vi "basic read field.vi"() -> (2 "Field":dbl[unit])   [LabVIEW 2012]
panel:
  in  "Read Field":bool
  in  "stop":bool
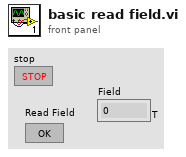
[diagram p1: front panel]
types:
  T1 = cluster{"function (0:volts DC)":u16, "range (0:auto)":u16, "rate (0:slow)":u16, "trigger mode (0:internal)":u16, "Autorange":bool}
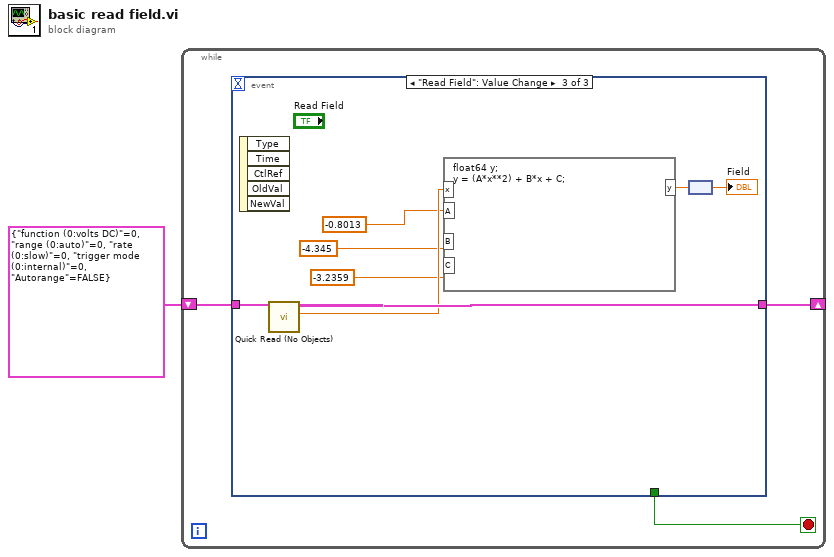
[diagram p0: block diagram]
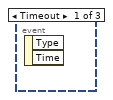
[diagram p2: hidden frame]
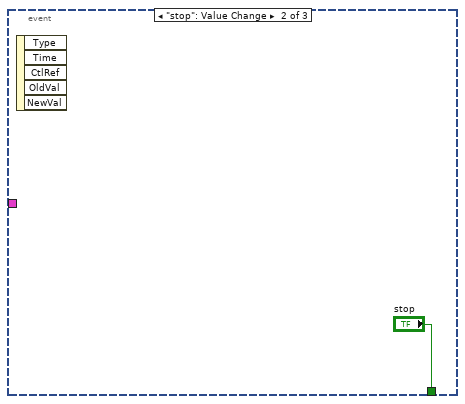
[diagram p3: hidden frame]
diagram:
  n1 = while {
    shift-right: [w2] -> _
    shift-left: T1 {"function (0:volts DC)"=0, "range (0:auto)"=0, "rate (0:slow)"=0, "trigger mode (0:internal)"=0, "Autorange"=FALSE} ("Fluke Multimeter In") -> [w3]
    stop <- w4 stop-if-true
    n2 = event shown="[2] \"Read Field\": Value Change" {
      selector: _ -> [_ _ _]
      dyn-events: _ -> [_ _ _]
      timeout: _ -> [_ _ _]
      tunnel: [_ "stop" _] -> w4
      tunnel: w3 -> [_ _ w13]
      tunnel: [_ _ w12] -> w2
      event Timeout {
        n3 = event-data() -> ()  [unwired: 1 in, 2 out]
      }
      event "stop": Value Change {
        n4 = event-data() -> ()  [unwired: 1 in, 5 out]
      }
      event "Read Field": Value Change {
        n5 = event-data() -> ()  [unwired: 1 in, 5 out]
        n6 = call "Quick Read (No Objects).vi"("Fluke Multimeter In"=w13) -> ("measurement"=w9:dbl, "Fluke Multimeter Out"=w12:T1)  [unwired: 7 in, 2 out]
        n7 = formula code="float64 y;\ny = (A*x**2) + B*x + C;"("x"=w9, "A"=-0.8013, "B"=-4.345, "C"=-3.2359) -> ("y"=w11:dbl)
        n8 = node(w11) -> (→"Field":dbl[unit])
      }
    }
  }
